vi "GetParam.vi"(8 "error in (no error)":errorcluster caption="entrée d'erreur (pas d'erreur)", 11 "Blobs.lvclass":refnum<class "Blobs.lvclass">) -> (0 "error out":errorcluster caption="sortie d'erreur", 2 "make_blobs":T1={"n_samples"=[100], "n_features"=2, "centers"=[], "cluster_std"=[], "centermin"=-10.0, "centermax"=10.0, "shuffle"=TRUE, "random_state"=-1, "Returns"="X"} {"random_state" min=-1; "n_features" min=1}, 3 "Blobs.lvclass":refnum<class "Blobs.lvclass">)   [LabVIEW 2020, in "Blobs.lvclass"]
doc: "Get Parameters"
uses:
  Blobs.lvclass
  Blobs.lvclass/Blobs.ctl
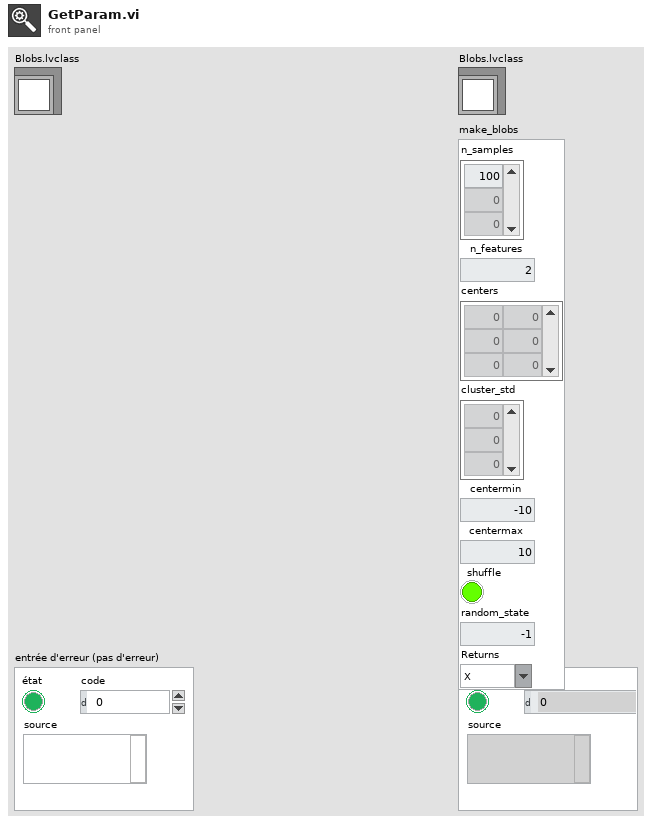
[diagram p1: front panel]
types:
  T1 = cluster{"n_samples":i32[], "n_features":u32, "centers":i32[][], "cluster_std":dbl[], "centermin":dbl, "centermax":dbl, "shuffle":bool, "random_state":i32, "Returns":string}
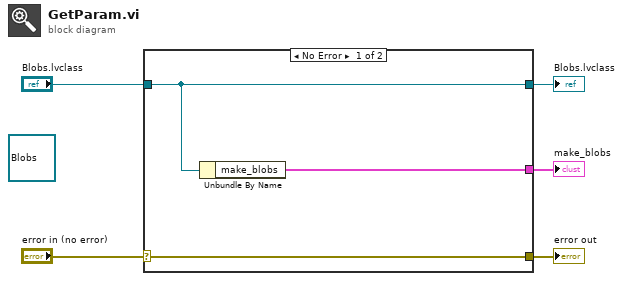
[diagram p0: block diagram]
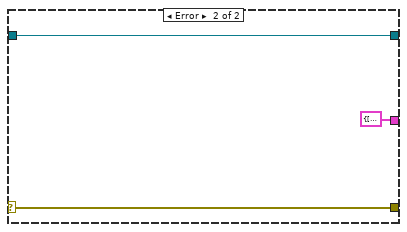
[diagram p2: hidden frame]
diagram:
  (unwired) refnum<class "Blobs.lvclass"> refnum ("Blobs.lvclass")
  n1 = case shown="No Error" "error in (no error)" {
    selector: "error in (no error)" -> [w8 w10]
    tunnel: [w8 w10] -> w4
    tunnel: [w7 w11] -> w2
    tunnel: "Blobs.lvclass" -> [w7 w11]
    tunnel: [w6 T1 {"n_samples"=[], "n_features"=0, "centers"=[], "cluster_std"=[], "centermin"=0.0, "centermax"=0.0, "shuffle"=FALSE, "random_state"=0, "Returns"=""} ("make_blobs")] -> w1
    frame No Error {
      n2 = Unbundle By Name(w7) -> ("make_blobs"=w6:T1)
    }
    frame Error {
    }
  }
  "error out" <- w4
  "Blobs.lvclass" <- w2
  "make_blobs" <- w1
